vi "InsertSubPanelViGen.vi"(8 "error in (no error)":errorcluster caption="entrée d'erreur (pas d'erreur)", 10 "RemVIRef":refnum<vi>, 11 "RemPanRef":refnum<vi>) -> (0 "sortie d'erreur":errorcluster, 2 "RemVIRefOut":refnum<vi>, 3 "RemPanRefOut":refnum<vi>)   [LabVIEW 2019]
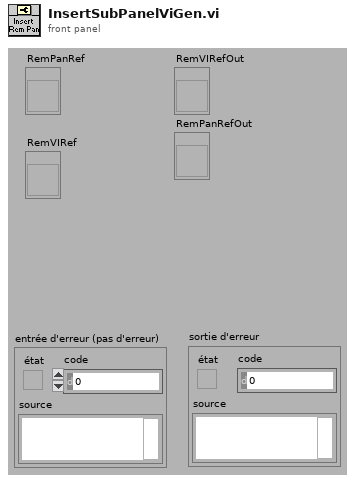
[diagram p1: front panel]
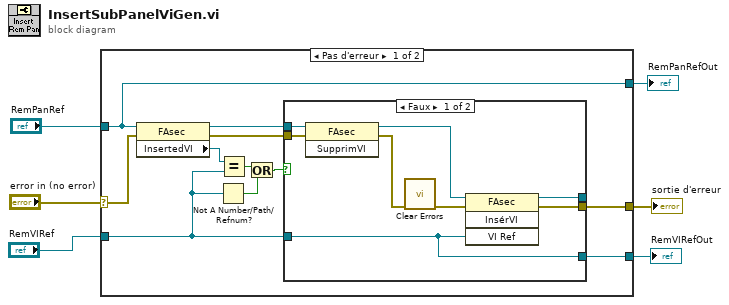
[diagram p0: block diagram]
diagram:
  n1 = case shown="Pas d'erreur" "error in (no error)" {
    selector: "error in (no error)" -> [w17 w29]
    tunnel: [w12 w29] -> w5
    tunnel: "RemPanRef" -> [w7 _]
    tunnel: "RemVIRef" -> [w9 _]
    tunnel: [w8 _] -> w2
    tunnel: [w7 _] -> w1
    frame No Error {
      n2 = property class="FAsec"(reference=w7, error in=w17) -> (reference out=w16:refnum<vi>, error out=w14:errorcluster, "InsertedVI"=w15:refnum<vi>)
      n3 = Not A Number/Path/Refnum?(number/path/refnum=w9) -> (NaN/Path/Refnum?=w10:bool)
      n4 = Equal?(x=w15, y=w9) -> (x = y?=w13:bool)
      n5 = Or(x=w13, y=w10) -> (x .or. y?=w11:bool)
      n6 = case shown="Faux" w11 {
        tunnel: w14 -> [w25 w28]
        tunnel: [w22 w28] -> w12
        tunnel: [w21 w27] -> _
        tunnel: w16 -> [w19 w27]
        tunnel: w9 -> [w18 w26]
        tunnel: [w18 w26] -> w8
        frame False {
          n7 = invoke on="Nœud de méthode" class="FAsec" method="SupprimVI"(reference=w19, error in=w25) -> (reference out=w24:refnum<vi>, error out=w23:errorcluster)  [unwired: 1 in, 1 out]
          n8 = call <vilib>:"Clear Errors.vi"("error in (no error)"=w23) -> ("error out"=w20:errorcluster)  [unwired: 5 in, 1 out]
          n9 = invoke on="Nœud de méthode" class="FAsec" method="InsérVI"(reference=w24, error in=w20, "VI Ref"=w18) -> (reference out=w21:refnum<vi>, error out=w22:errorcluster)  [unwired: 1 in, 2 out]
        }
        frame True {
          # "Vi Already In"
        }
      }
    }
    frame Error {
    }
  }
  "sortie d'erreur" <- w5
  "RemVIRefOut" <- w2
  "RemPanRefOut" <- w1
